vi "ExecuteXML.vi"(8 "error in (no error)":errorcluster, 11 "Auto File Path":path=path "C:/Users/Bendethic/Desktop/AutoRoutineCreator/AutoFiles/1A.txt") -> (0 "error out":errorcluster)   [LabVIEW 2017]
uses:
  RoutineData.vi
panel:
  in  "Boolean":bool
  out "XML String":string
  out "Routine Data":T1
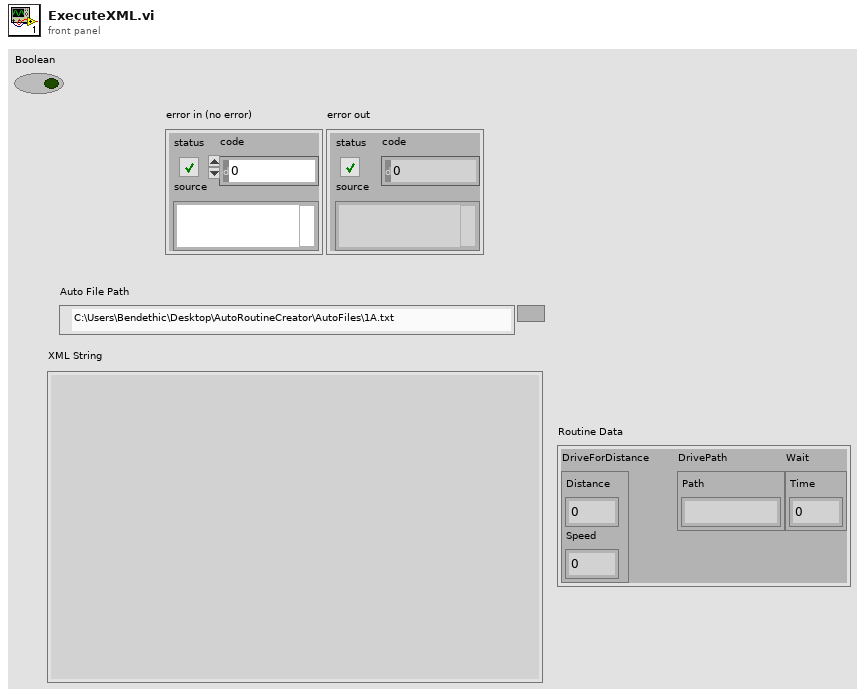
[diagram p1: front panel]
types:
  T1 = cluster{"DriveForDistance":cluster{"Distance":dbl, "Speed":dbl}, "DrivePath":cluster{"Path":string}, "Wait":cluster{"Time":u32}}
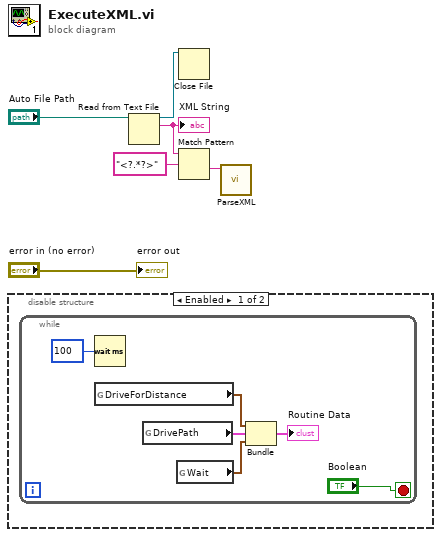
[diagram p0: block diagram]
diagram:
  n1 = disable-structure shown="Enabled" {
    frame Enabled {
      n2 = while {
        stop <- "Boolean" stop-if-true
        n3 = Wait (ms)(milliseconds to wait=u32 100) -> ()  [unwired: 1 out]
        n4 = global read "RoutineData.vi" "DriveForDistance"() -> (w11:cluster{"Distance":dbl, "Speed":dbl})
        n5 = global read "RoutineData.vi" "DrivePath"() -> (w10:cluster{"Path":string})
        n6 = global read "RoutineData.vi" "Wait"() -> (w9:cluster{"Time":u32})
        n7 = Bundle("DriveForDistance"=w11, "DrivePath"=w10, "Wait"=w9) -> (→"Routine Data":T1)  [unwired: 1 in]
      }
    }
    frame Disabled {
    }
  }
  n8 = Read from Text File(file (use dialog)="Auto File Path") -> (refnum out=w3:refnum<file>, text=w4:string)  [unwired: 3 in, 2 out]
  "XML String" <- w4
  n9 = Close File(refnum=w3) -> ()  [unwired: 1 in, 2 out]
  n10 = Match Pattern(string=w4, regular expression="<?.*?>") -> (after substring=w2:string)  [unwired: 1 in, 3 out]
  n11 = call "ParseXML.vi"("Node"=w2) -> ()  [unwired: 10 in, 1 out]
  "error out" <- "error in (no error)"
